vi "串口自动测试.vi"(9 "RS485选择":bool, 11 "RS232选择":bool) -> ()   [LabVIEW 2010]
uses:
  <vilib>/Instr/_visa.llb/VISA Configure Serial Port (Instr).vi
  全局量/试验配置信息.vi
  全局量/自动测试结果.vi
panel:
  in  "第2路RS485":string
  in  "第1路RS485":string
  in  "第2路RS232":string
  in  "第1路RS232":string
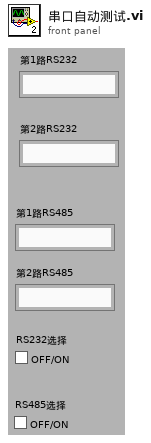
[diagram p1: front panel]
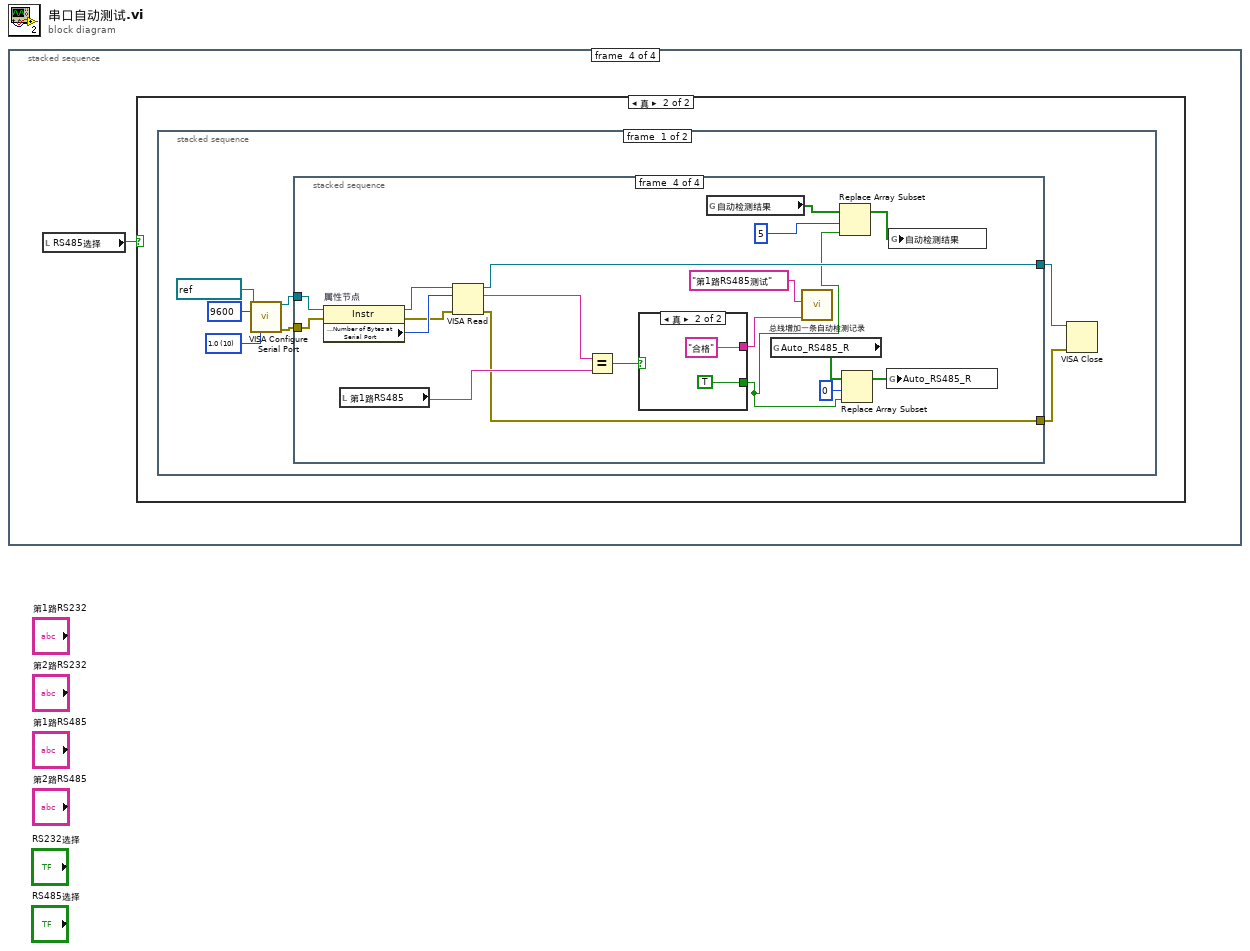
[diagram p0: block diagram]
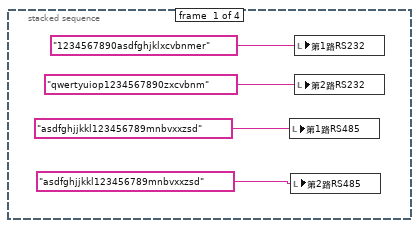
[diagram p2: hidden frame]
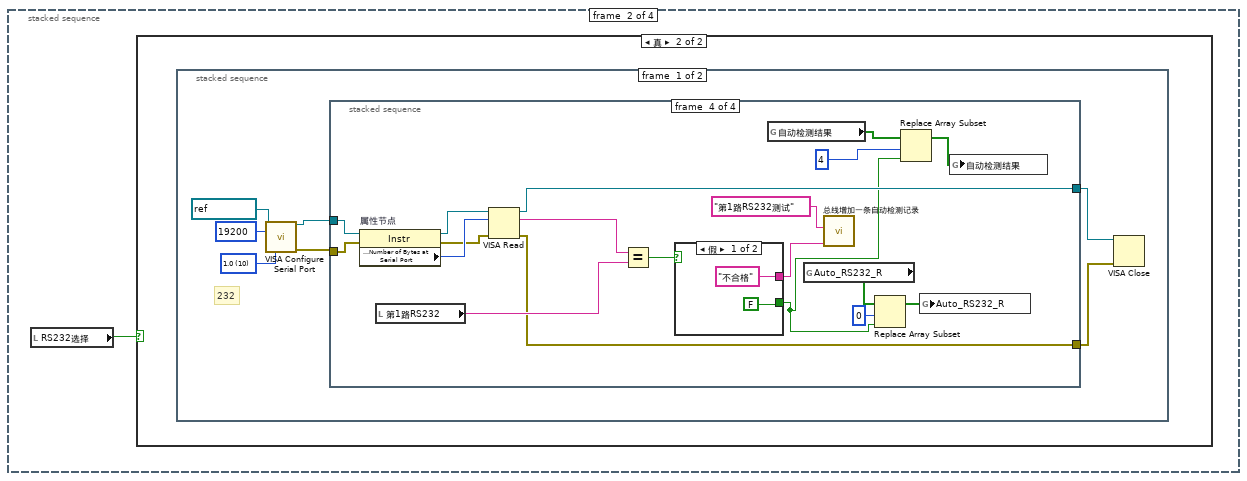
[diagram p3: hidden frame]
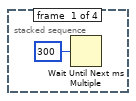
[diagram p5: hidden frame]
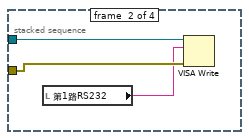
[diagram p6: hidden frame]
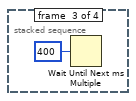
[diagram p7: hidden frame]
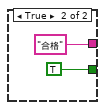
[diagram p8: hidden frame]
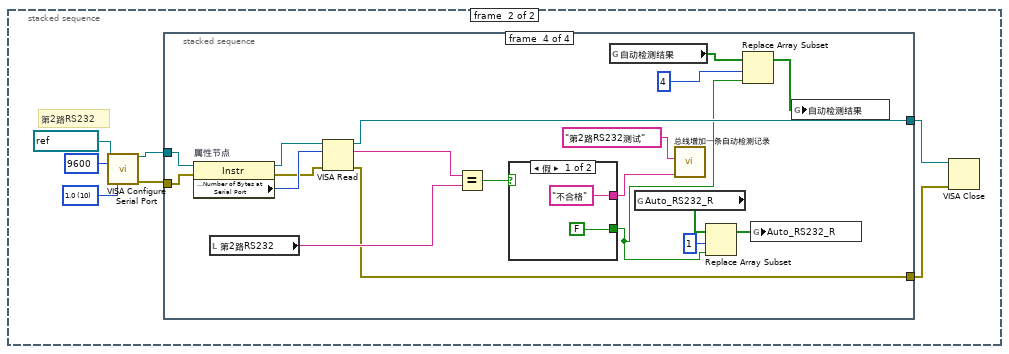
[diagram p9: hidden frame]
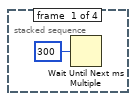
[diagram p10: hidden frame]
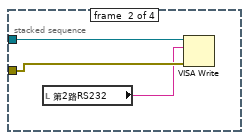
[diagram p11: hidden frame]
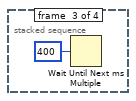
[diagram p12: hidden frame]
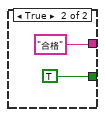
[diagram p13: hidden frame]
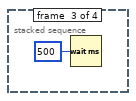
[diagram p14: hidden frame]
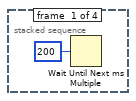
[diagram p16: hidden frame]
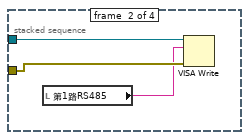
[diagram p17: hidden frame]
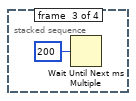
[diagram p18: hidden frame]
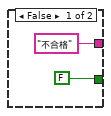
[diagram p19: hidden frame]
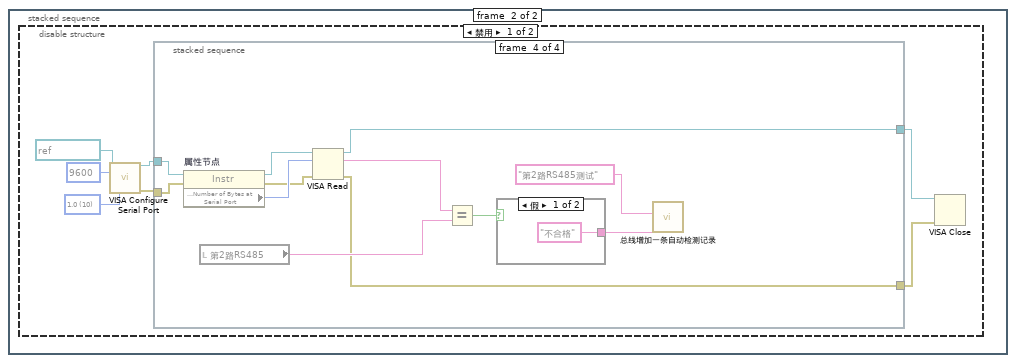
[diagram p20: hidden frame]
diagram:
  n1 = stacked-sequence {
    frame #0 {
      n2 = local write "第1路RS485"("asdfghjjkkl123456789mnbvxxzsd" ("发送字符串_3")) -> ()
      n3 = local write "第2路RS485"("asdfghjjkkl123456789mnbvxxzsd" ("发送字符串_3")) -> ()
      n4 = local write "第1路RS232"("1234567890asdfghjklxcvbnmer" ("发送字符串_1")) -> ()
      n5 = local write "第2路RS232"("qwertyuiop1234567890zxcvbnm" ("发送字符串_2")) -> ()
    }
    frame #1 {
      n6 = local read "RS232选择"() -> (w5:bool)
      n7 = case shown="真" w5 {
        frame False {
        }
        frame True {
          n8 = stacked-sequence {
            frame #0 {
              w8 = u16 10 items=["1.0"=10, "1.5"=15, "2.0"=20] ("stop bits (10: 1 bit)")
              # "232"
              n9 = call-poly "VISA Configure Serial Port"("VISA resource name"=refnum<visa-resource-name> "COM1", "baud rate (9600)"=u32 19200, "stop bits (10: 1 bit)"=w8) -> ("VISA resource name out"=w7:refnum<visa-resource-name>, "error out"=w6:errorcluster)  [unwired: 11 in]
              n10 = stacked-sequence {
                tunnel: w7 -> [_ w16 _ w29]
                tunnel: w6 -> [_ w15 _ w28]
                tunnel: [_ _ _ w31] -> w12
                tunnel: [_ _ _ w30] -> w11
                frame #0 {
                  n11 = Wait Until Next ms Multiple(millisecond multiple=u32 300 ("毫秒倍数")) -> ()  [unwired: 1 out]
                }
                frame #1 {
                  n12 = local read "第1路RS232"() -> (w14:string)
                  n13 = VISA Write(VISA resource name=w16, write buffer=w14, error in (no error)=w15) -> ()  [unwired: 3 out]
                }
                frame #2 {
                  n14 = Wait Until Next ms Multiple(millisecond multiple=u32 400 ("毫秒倍数")) -> ()  [unwired: 1 out]
                }
                frame #3 {
                  n15 = property on="属性节点" class="Instr"(reference=w29, error in=w28) -> (reference out=w35:refnum<visa-resource-name>, error out=w33:errorcluster, "Serial Settings:Number of Bytes at Serial Port"=w34:u32)
                  n16 = local read "第1路RS232"() -> (w32:string)
                  n17 = VISA Read(VISA resource name=w35, byte count=w34, error in (no error)=w33) -> (VISA resource name out=w31:refnum<visa-resource-name>, read buffer=w27:string, error out=w30:errorcluster)  [unwired: 1 out]
                  n18 = Equal?(x=w27, y=w32) -> (x = y?=w36:bool)
                  n19 = case shown="假" w36 {
                    tunnel: ["不合格" "合格"] -> w25
                    tunnel: [FALSE TRUE] -> w18
                    frame False {
                    }
                    frame True {
                    }
                  }
                  n20 = global read "试验配置信息.vi" "自动检测结果"() -> (w19:bool[])
                  n21 = global read "自动测试结果.vi" "Auto_RS232_R"() -> (w24:bool[])
                  n22 = call "总线增加一条自动检测记录.vi"("测试结果"=w25, "测试内容"="第1路RS232测试") -> ()  [unwired: 10 in]
                  n23 = Replace Array Subset(array=w24, new element=w18, index=0 ("索引")) -> (w23:bool[])
                  n24 = Replace Array Subset(array=w19, new element=w18, index=4 ("索引")) -> (w20:bool[])
                  n25 = global write "自动测试结果.vi" "Auto_RS232_R"(w23) -> ()
                  n26 = global write "试验配置信息.vi" "自动检测结果"(w20) -> ()
                }
              }
              n27 = VISA Close(VISA resource name=w12, error in (no error)=w11) -> ()  [unwired: 1 out]
            }
            frame #1 {
              w43 = u16 10 items=["1.0"=10, "1.5"=15, "2.0"=20] ("stop bits (10: 1 bit)")
              # "第2路RS232"
              n28 = call-poly "VISA Configure Serial Port"("VISA resource name"=refnum<visa-resource-name> "COM3", "baud rate (9600)"=u32 9600, "stop bits (10: 1 bit)"=w43) -> ("VISA resource name out"=w46:refnum<visa-resource-name>, "error out"=w47:errorcluster)  [unwired: 11 in]
              n29 = stacked-sequence {
                tunnel: w46 -> [_ w51 _ w64]
                tunnel: w47 -> [_ w50 _ w63]
                tunnel: [_ _ _ w66] -> w41
                tunnel: [_ _ _ w65] -> w42
                frame #0 {
                  n30 = Wait Until Next ms Multiple(millisecond multiple=u32 300 ("毫秒倍数")) -> ()  [unwired: 1 out]
                }
                frame #1 {
                  n31 = local read "第2路RS232"() -> (w49:string)
                  n32 = VISA Write(VISA resource name=w51, write buffer=w49, error in (no error)=w50) -> ()  [unwired: 3 out]
                }
                frame #2 {
                  n33 = Wait Until Next ms Multiple(millisecond multiple=u32 400 ("毫秒倍数")) -> ()  [unwired: 1 out]
                }
                frame #3 {
                  n34 = property on="属性节点" class="Instr"(reference=w64, error in=w63) -> (reference out=w70:refnum<visa-resource-name>, error out=w68:errorcluster, "Serial Settings:Number of Bytes at Serial Port"=w69:u32)
                  n35 = local read "第2路RS232"() -> (w67:string)
                  n36 = VISA Read(VISA resource name=w70, byte count=w69, error in (no error)=w68) -> (VISA resource name out=w66:refnum<visa-resource-name>, read buffer=w60:string, error out=w65:errorcluster)  [unwired: 1 out]
                  n37 = Equal?(x=w60, y=w67) -> (x = y?=w71:bool)
                  n38 = case shown="假" w71 {
                    tunnel: ["不合格" "合格"] -> w61
                    tunnel: [FALSE TRUE] -> w53
                    frame False {
                    }
                    frame True {
                    }
                  }
                  n39 = global read "试验配置信息.vi" "自动检测结果"() -> (w54:bool[])
                  n40 = global read "自动测试结果.vi" "Auto_RS232_R"() -> (w59:bool[])
                  n41 = call "总线增加一条自动检测记录.vi"("测试结果"=w61, "测试内容"="第2路RS232测试") -> ()  [unwired: 10 in]
                  n42 = Replace Array Subset(array=w59, new element=w53, index=1 ("索引")) -> (w58:bool[])
                  n43 = Replace Array Subset(array=w54, new element=w53, index=4 ("索引")) -> (w55:bool[])
                  n44 = global write "自动测试结果.vi" "Auto_RS232_R"(w58) -> ()
                  n45 = global write "试验配置信息.vi" "自动检测结果"(w55) -> ()
                }
              }
              n46 = VISA Close(VISA resource name=w41, error in (no error)=w42) -> ()  [unwired: 1 out]
            }
          }
        }
      }
    }
    frame #2 {
      n47 = Wait (ms)(milliseconds to wait=u32 500 ("等待时间（毫秒）")) -> ()  [unwired: 1 out]
    }
    frame #3 {
      n48 = local read "RS485选择"() -> (w77:bool)
      n49 = case shown="真" w77 {
        frame False {
        }
        frame True {
          n50 = stacked-sequence {
            frame #0 {
              w82 = u16 10 items=["1.0"=10, "1.5"=15, "2.0"=20] ("stop bits (10: 1 bit)")
              n51 = call-poly "VISA Configure Serial Port"("VISA resource name"=refnum<visa-resource-name> "COM4", "baud rate (9600)"=u32 9600, "stop bits (10: 1 bit)"=w82) -> ("VISA resource name out"=w79:refnum<visa-resource-name>, "error out"=w78:errorcluster)  [unwired: 11 in]
              n52 = stacked-sequence {
                tunnel: w79 -> [_ w88 _ w101]
                tunnel: w78 -> [_ w87 _ w100]
                tunnel: [_ _ _ w103] -> w84
                tunnel: [_ _ _ w102] -> w83
                frame #0 {
                  n53 = Wait Until Next ms Multiple(millisecond multiple=u32 200 ("毫秒倍数")) -> ()  [unwired: 1 out]
                }
                frame #1 {
                  n54 = local read "第1路RS485"() -> (w86:string)
                  n55 = VISA Write(VISA resource name=w88, write buffer=w86, error in (no error)=w87) -> ()  [unwired: 3 out]
                }
                frame #2 {
                  n56 = Wait Until Next ms Multiple(millisecond multiple=u32 200 ("毫秒倍数")) -> ()  [unwired: 1 out]
                }
                frame #3 {
                  n57 = property on="属性节点" class="Instr"(reference=w101, error in=w100) -> (reference out=w107:refnum<visa-resource-name>, error out=w105:errorcluster, "Serial Settings:Number of Bytes at Serial Port"=w106:u32)
                  n58 = local read "第1路RS485"() -> (w104:string)
                  n59 = VISA Read(VISA resource name=w107, byte count=w106, error in (no error)=w105) -> (VISA resource name out=w103:refnum<visa-resource-name>, read buffer=w99:string, error out=w102:errorcluster)  [unwired: 1 out]
                  n60 = Equal?(x=w99, y=w104) -> (x = y?=w108:bool)
                  n61 = case shown="真" w108 {
                    tunnel: ["不合格" "合格"] -> w97
                    tunnel: [FALSE TRUE] -> w90
                    frame False {
                    }
                    frame True {
                    }
                  }
                  n62 = global read "试验配置信息.vi" "自动检测结果"() -> (w91:bool[])
                  n63 = global read "自动测试结果.vi" "Auto_RS485_R"() -> (w96:bool[])
                  n64 = call "总线增加一条自动检测记录.vi"("测试结果"=w97, "测试内容"="第1路RS485测试") -> ()  [unwired: 10 in]
                  n65 = Replace Array Subset(array=w91, new element=w90, index=5 ("索引")) -> (w92:bool[])
                  n66 = Replace Array Subset(array=w96, new element=w90, index=0 ("索引")) -> (w95:bool[])
                  n67 = global write "自动测试结果.vi" "Auto_RS485_R"(w95) -> ()
                  n68 = global write "试验配置信息.vi" "自动检测结果"(w92) -> ()
                }
              }
              n69 = VISA Close(VISA resource name=w84, error in (no error)=w83) -> ()  [unwired: 1 out]
            }
            frame #1 {
              n70 = disable-structure shown="禁用" {
                frame Disabled {
                  w119 = u16 10 items=["1.0"=10, "1.5"=15, "2.0"=20] ("stop bits (10: 1 bit)")
                  n71 = call-poly "VISA Configure Serial Port"("VISA resource name"=refnum<visa-resource-name> "COM5", "baud rate (9600)"=u32 9600, "stop bits (10: 1 bit)"=w119) -> ("VISA resource name out"=w114:refnum<visa-resource-name>, "error out"=w113:errorcluster)  [unwired: 11 in]
                  n72 = stacked-sequence {
                    tunnel: w114 -> [_ w123 _ w129]
                    tunnel: w113 -> [_ w122 _ w128]
                    tunnel: [_ _ _ w131] -> w116
                    tunnel: [_ _ _ w130] -> w115
                    frame #0 {
                      n73 = Wait Until Next ms Multiple(millisecond multiple=u32 200 ("毫秒倍数")) -> ()  [unwired: 1 out]
                    }
                    frame #1 {
                      n74 = local read "第2路RS485"() -> (w121:string)
                      n75 = VISA Write(VISA resource name=w123, write buffer=w121, error in (no error)=w122) -> ()  [unwired: 3 out]
                    }
                    frame #2 {
                      n76 = Wait Until Next ms Multiple(millisecond multiple=u32 200 ("毫秒倍数")) -> ()  [unwired: 1 out]
                    }
                    frame #3 {
                      n77 = property on="属性节点" class="Instr"(reference=w129, error in=w128) -> (reference out=w135:refnum<visa-resource-name>, error out=w133:errorcluster, "Serial Settings:Number of Bytes at Serial Port"=w134:u32)
                      n78 = local read "第2路RS485"() -> (w132:string)
                      n79 = VISA Read(VISA resource name=w135, byte count=w134, error in (no error)=w133) -> (VISA resource name out=w131:refnum<visa-resource-name>, read buffer=w127:string, error out=w130:errorcluster)  [unwired: 1 out]
                      n80 = Equal?(x=w127, y=w132) -> (x = y?=w136:bool)
                      n81 = case shown="假" w136 {
                        tunnel: ["不合格" "合格"] -> w125
                        frame False {
                        }
                        frame True {
                        }
                      }
                      n82 = call "总线增加一条自动检测记录.vi"("测试结果"=w125, "测试内容"="第2路RS485测试") -> ()  [unwired: 10 in]
                    }
                  }
                  n83 = VISA Close(VISA resource name=w116, error in (no error)=w115) -> ()  [unwired: 1 out]
                }
                frame Enabled {
                }
              }
            }
          }
        }
      }
    }
  }
